vi "AuMT8852B EDR Differential Phase Encoding Results.vi"(8 "error in (no error)":errorcluster, 11 "VISA session":refnum<visa-resource-name>) -> (0 "error out":errorcluster, 2 "error code":i32, 3 "VISA session out":refnum<visa-resource-name>, 4 "Results":T1)   [LabVIEW 2017]
doc: "Anritsu MT8852B Bluetooth Tester\n\nReturns the summary results of the EDR Differential Phase Encoding test.\n\nOUTPUT\nResults - measurements made during the test."
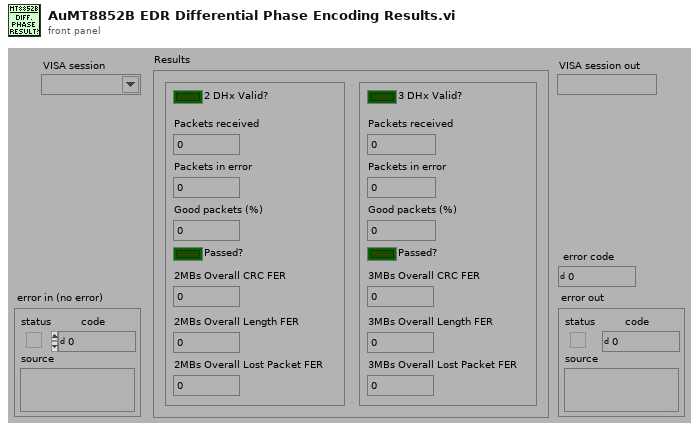
[diagram p1: front panel]
types:
  T1 = cluster{"2 DHx Valid?":bool, "Packets received":u32, "Packets in error":u32, "Passed?":bool, "Good packets (%)":u32, "3 DHx Valid?":bool, "Packets received":u32, "Packets in error":u32, "Passed?":bool, "Good packets (%)":u32, "2MBs Overall CRC FER":u32, "2MBs Overall Length FER":u32, "2MBs Overall Lost Packet FER":u32, "3MBs Overall CRC FER":u32, "3MBs Overall Length FER":u32, "3MBs Overall Lost Packet FER":u32}
  T2 = enum16{"Simulate", "Range check", "Cache", "Query instrument status"}
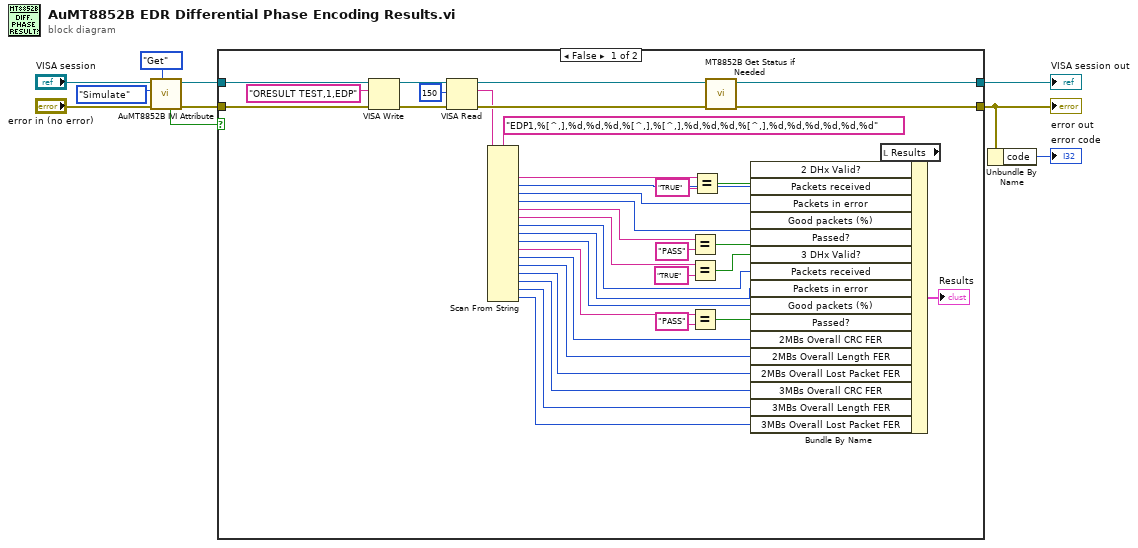
[diagram p0: block diagram]
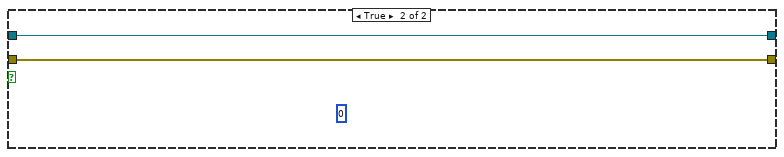
[diagram p2: hidden frame]
diagram:
  n1 = call <instrlib>:"AuMT8852B IVI Attribute.vi"("Set/Get (Set)"=enum16{"Set", "Get"}."Get", "error in (no error)"="error in (no error)", "Flag (Simulate)"=T2."Simulate", "VISA session"="VISA session") -> ("error out"=w7:errorcluster, "VISA session out"=w9:refnum<visa-resource-name>, "Value out"=w3:bool)  [unwired: 5 in]
  n2 = case shown="False" w3 {
    tunnel: [w40 w50] -> w10
    tunnel: [w39 w49] -> w1
    tunnel: w9 -> [w47 w50]
    tunnel: w7 -> [w46 w49]
    frame False {
      n3 = VISA Write(VISA resource name=w47, write buffer="ORESULT TEST,1,EDP" ("write buffer (\"\")"), error in (no error)=w46) -> (VISA resource name out=w45:refnum<visa-resource-name>, error out=w44:errorcluster)  [unwired: 1 out]
      n4 = VISA Read(VISA resource name=w45, byte count=u32 150 ("byte count (0)"), error in (no error)=w44) -> (VISA resource name out=w38:refnum<visa-resource-name>, read buffer=w36:string, error out=w37:errorcluster)  [unwired: 1 out]
      n5 = Scan From String(format string="EDP1,%[^,],%d,%d,%d,%[^,],%[^,],%d,%d,%d,%[^,],%d,%d,%d,%d,%d,%d" ("Format String"), input string=w36) -> (output 1=w35:string, output 2=w31:i32, output 3=w30:i32, output 4=w29:i32, output 5=w26:string, output 6=w23:string, output 7=w22:i32, output 8=w21:i32, output 9=w20:i32, output 10=w19:string, output 11=w16:i32, output 12=w15:i32, output 13=w14:i32, output 14=w13:i32, output 15=w12:i32, output 16=w11:i32)  [unwired: 18 in, 3 out]
      n6 = Equal?(x=w26, y="PASS") -> (x = y?=w25:bool)
      n7 = Equal?(x=w23, y="TRUE") -> (x = y?=w24:bool)
      n8 = Equal?(x=w19, y="PASS") -> (x = y?=w18:bool)
      n9 = Equal?(x=w35, y="TRUE") -> (x = y?=w32:bool)
      n10 = call <instrlib>:"MT8852B Get Status if Needed.vi"("error in (no error)"=w37, "VISA session"=w38) -> ("error out"=w39:errorcluster, "VISA session out"=w40:refnum<visa-resource-name>)  [unwired: 8 in]
      n11 = local read "Results"() -> (w33:T1)
      n12 = Bundle By Name(cluster=w33, "2 DHx Valid?"=w32, "Packets received"=w31, "Packets in error"=w30, "Good packets (%)"=w29, "Passed?"=w25, "3 DHx Valid?"=w24, "Packets received"=w22, "Packets in error"=w21, "Good packets (%)"=w20, "Passed?"=w18, "2MBs Overall CRC FER"=w16, "2MBs Overall Length FER"=w15, "2MBs Overall Lost Packet FER"=w14, "3MBs Overall CRC FER"=w13, "3MBs Overall Length FER"=w12, "3MBs Overall Lost Packet FER"=w11) -> (→"Results":T1)
    }
    frame True {
      (unwired) u8 0
    }
  }
  "error out" <- w1
  "VISA session out" <- w10
  n13 = Unbundle By Name(w1) -> ("code"=→"error code":i32)
